vi "Release Agent Public Key.vi"(8 "error in (no error)":errorcluster, 11 "agent public key":T1) -> (0 "error out":errorcluster)   [LabVIEW 2017, in "libssh2.lvlib"]
doc: "Release the memory associated with an agent public key."
uses:
  libssh2.lvlib
  Agent Public Key Refnum.ctl
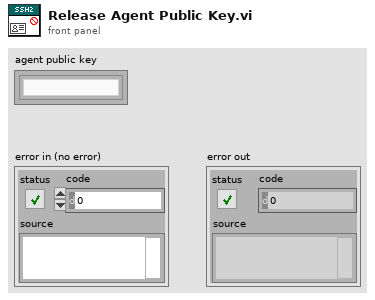
[diagram p1: front panel]
types:
  T1 = typedef "libssh2.lvlib/Agent Public Key Refnum.ctl" = refnum<k1>
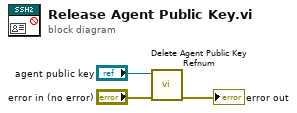
[diagram p0: block diagram]
diagram:
  n1 = call "Delete Agent Public Key Refnum.vi"("error in (no error)"="error in (no error)", "agent public key"="agent public key") -> ("error out"=→"error out":errorcluster)  [unwired: 8 in, 1 out]
